vi "EXAM_YV9K29-(WITH CLUSTER).vi"() -> ()   [LabVIEW 2021]
panel:
  in  "Cluster":T1
  in  "OK Button":bool
  out "text":string
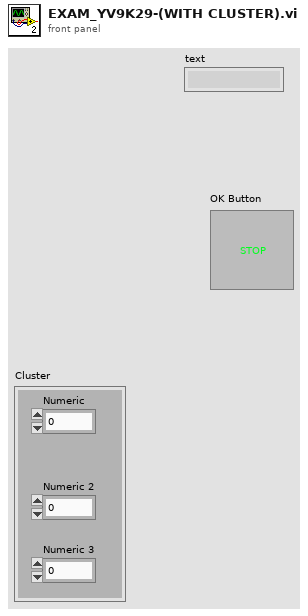
[diagram p1: front panel]
types:
  T1 = cluster{"Numeric":dbl, "Numeric 2":dbl, "Numeric 3":dbl}
  T2 = enum16{"open", "replace", "create", "open or create", "replace or create", "replace or create with confirmation"}
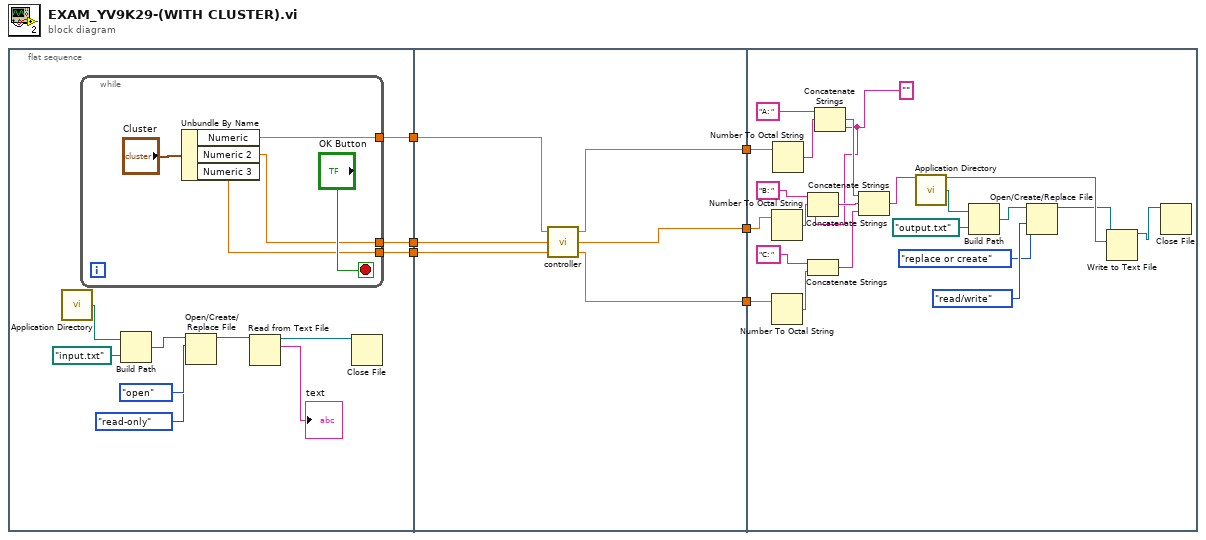
[diagram p0: block diagram]
diagram:
  n1 = flat-sequence {
    tunnel: [w9] -> w3
    tunnel: [w8] -> w2
    tunnel: [w7] -> w1
    tunnel: [w28] -> w6
    tunnel: [w27] -> w5
    tunnel: [w26] -> w4
    tunnel: w3 -> [w25]
    tunnel: w2 -> [w24]
    tunnel: w1 -> [w23]
    tunnel: w6 -> [w33]
    tunnel: w5 -> [w32]
    tunnel: w4 -> [w31]
    frame #0 {
      n2 = call <vilib>:"Application Directory.vi"() -> ("Application Directory"=w16:path)
      n3 = while {
        tunnel: [w20] -> w9
        tunnel: [w19] -> w8
        tunnel: [w18] -> w7
        stop <- "OK Button" stop-if-true
        n4 = Unbundle By Name("Cluster") -> ("Numeric"=w20:dbl, "Numeric 2"=w19:dbl, "Numeric 3"=w18:dbl)
      }
      n5 = Build Path(base path=w16, name or relative path=path "input.txt") -> (appended path=w14:path)
      n6 = Open/Create/Replace File(file path (use dialog)=w14, operation (0:open)=T2."open", access (0:read/write)=enum16{"read/write", "read-only", "write-only"}."read-only") -> (refnum out=w10:refnum<file>)  [unwired: 3 in, 2 out]
      n7 = Read from Text File(file (use dialog)=w10) -> (refnum out=w17:refnum<file>, text=→"text":string)  [unwired: 3 in, 2 out]
      n8 = Close File(refnum=w17) -> ()  [unwired: 1 in, 2 out]
    }
    frame #1 {
      n9 = call "controller.vi"("Number C"=w23, "Number B"=w24, "Number A"=w25) -> ("RESULT B"=w26:dbl, "RESULT C"=w27:dbl, "RESULT A"=w28:dbl)
    }
    frame #2 {
      w30 = "" ("string")
      n10 = Number To Octal String(2:w32) -> (0:w49:string)  [unwired: 1 in]
      n11 = Number To Octal String(2:w31) -> (0:w48:string)  [unwired: 1 in]
      n12 = Number To Octal String(2:w33) -> (0:w43:string)  [unwired: 1 in]
      n13 = Concatenate Strings("B: " ("string"), w49, w30) -> (w45:string)
      n14 = Concatenate Strings("C: " ("string"), w48) -> (w46:string)
      n15 = Concatenate Strings("A: ", w43, w30) -> (w44:string)
      n16 = Concatenate Strings(w44, w45, w46) -> (w47:string)
      n17 = call <vilib>:"Application Directory.vi"() -> ("Application Directory"=w41:path)
      n18 = Build Path(base path=w41, name or relative path=path "output.txt") -> (appended path=w40:path)
      n19 = Open/Create/Replace File(file path (use dialog)=w40, operation (0:open)=T2."replace or create", access (0:read/write)=enum16{"read/write", "read-only", "write-only"}."read/write") -> (refnum out=w42:refnum<file>)  [unwired: 3 in, 2 out]
      n20 = Write to Text File(file (use dialog)=w42, text=w47) -> (refnum out=w29:refnum<file>)  [unwired: 2 in, 2 out]
      n21 = Close File(refnum=w29) -> ()  [unwired: 1 in, 2 out]
    }
  }
